vi "myRIO_BRig_RT__Case_Exp_State_initTrial_LC_ENL1.vi"(6 "input_dataTrial":u16[][](array[numeric]), 7 "input_spout":enum16{"Left", "Right"}(ring), 9 "input_dataBlock":u16[][](array[numeric]), 10 "input_dataLC":u16[](array[numeric]), 11 "input_dataCurrent":u16[](array[numeric])) -> (2 "output_LC__ENL1":bool, 3 "output_LC_led__ENL1":bool, 4 "output_dataTrial":u16[][](array[numeric]), 5 "output_dataCurrent":u16[](array[numeric]))   [LabVIEW 2014]
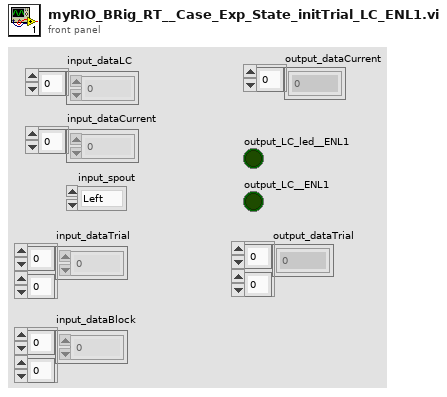
[diagram p1: front panel]
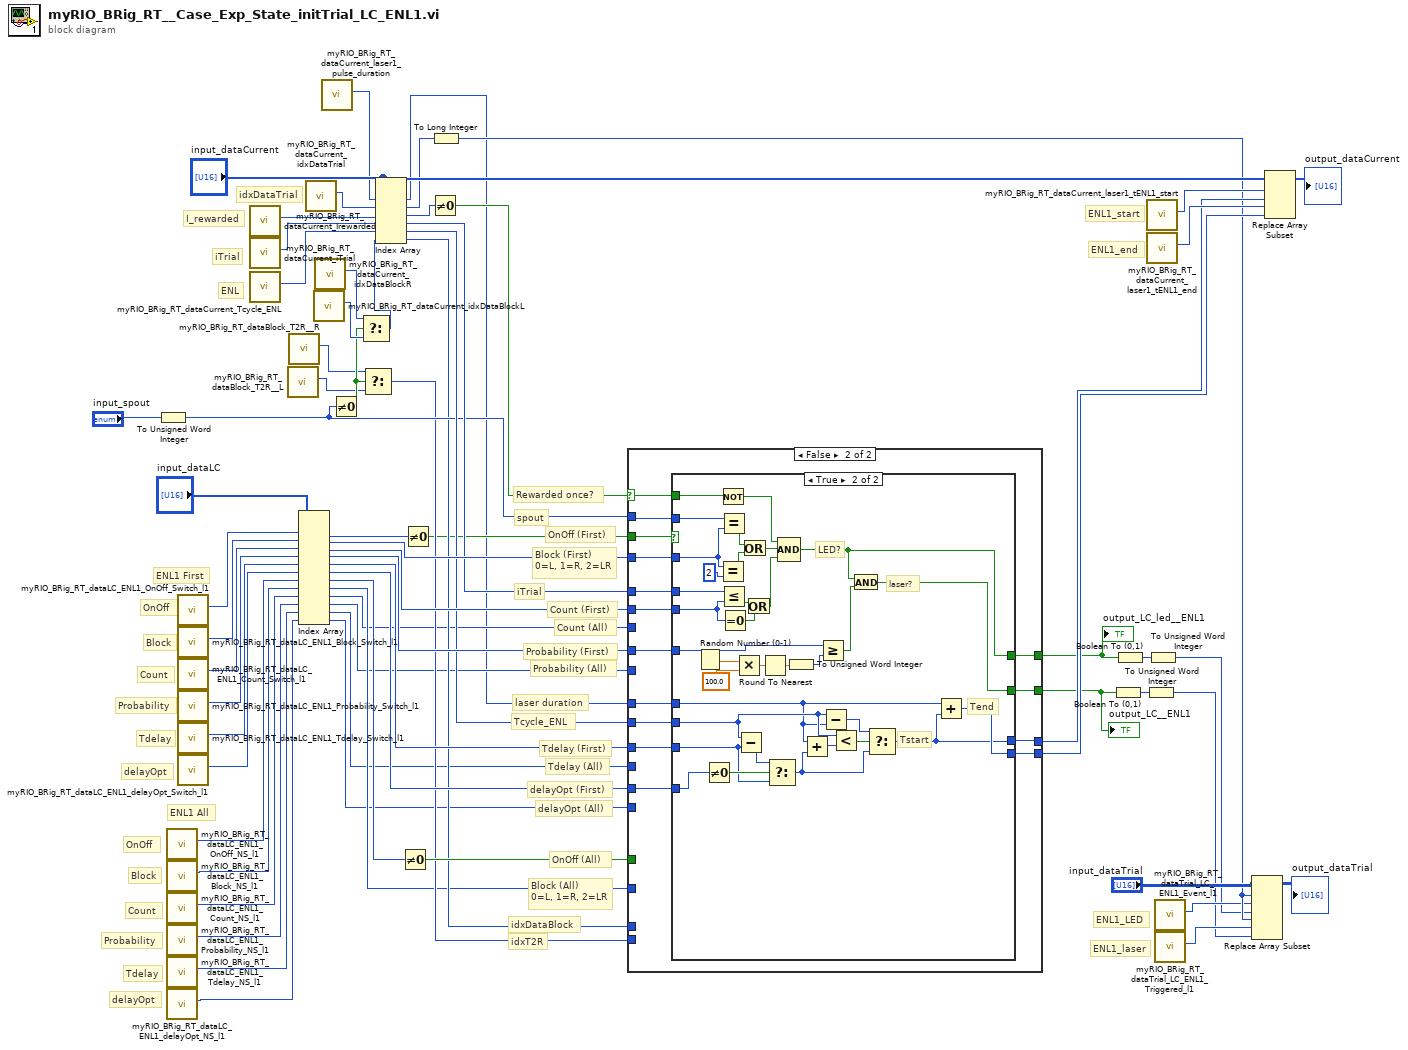
[diagram p0: block diagram]
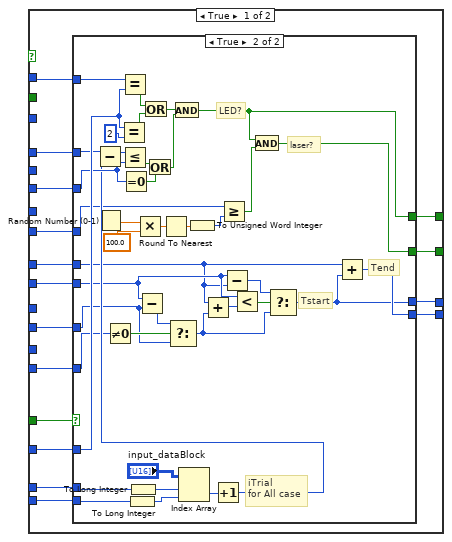
[diagram p2: hidden frame]
diagram:
  # "delayOpt (All)"
  # "Tdelay (All)"
  # "Probability (All)"
  # "Count (All)"
  # "Block (All)\n0=L, 1=R, 2=LR"
  # "idxT2R"
  # "idxDataBlock"
  # "OnOff (All)"
  # "delayOpt"
  # "Count"
  # "Tdelay"
  # "Probability"
  # "OnOff"
  # "Block"
  # "ENL1 All"
  # "Tdelay (First)"
  # "delayOpt (First)"
  # "Tcycle_ENL"
  # "laser duration"
  # "Probability (First)"
  # "Count (First)"
  # "iTrial"
  # "Block (First)\n0=L, 1=R, 2=LR"
  # "spout"
  # "Rewarded once?"
  # "OnOff (First)"
  # "iTrial"
  # "ENL1_LED"
  # "ENL1_laser"
  # "idxDataTrial"
  # "ENL1_end"
  # "ENL1_start"
  # "delayOpt"
  # "ENL"
  # "Tdelay"
  # "I_rewarded"
  # "ENL1 First"
  # "Probability"
  # "Count"
  # "Block"
  # "OnOff"
  n1 = To Unsigned Word Integer(number="input_spout") -> (unsigned 16bit integer=w24:u16)
  n2 = call "myRIO_BRig_RT_dataLC_ENL1_OnOff_NS_l1.vi"() -> ("output_ENL1_OnOff_NS_l1"=w10:i32)  [unwired: 11 in]
  n3 = call "myRIO_BRig_RT_dataLC_ENL1_Block_NS_l1.vi"() -> ("output_ENL1_All_Block"=w9:i32)  [unwired: 11 in]
  n4 = call "myRIO_BRig_RT_dataLC_ENL1_Count_NS_l1.vi"() -> ("output_ENL1_Count_NS_l1"=w8:i32)  [unwired: 11 in]
  n5 = call "myRIO_BRig_RT_dataLC_ENL1_Probability_NS_l1.vi"() -> ("output_ENL1_Probability_NS_l1"=w7:i32)  [unwired: 11 in]
  n6 = call "myRIO_BRig_RT_dataLC_ENL1_Tdelay_NS_l1.vi"() -> ("output_ENL1_Tdelay_NS_l1"=w6:i32)  [unwired: 11 in]
  n7 = call "myRIO_BRig_RT_dataLC_ENL1_delayOpt_NS_l1.vi"() -> ("output_ENL1_delayOpt_NS_l1"=w5:i32)  [unwired: 11 in]
  n8 = call "myRIO_BRig_RT_dataLC_ENL1_OnOff_Switch_l1.vi"() -> ("output_ENL1_OnOff_Switch_l1"=w64:i32)  [unwired: 11 in]
  n9 = call "myRIO_BRig_RT_dataLC_ENL1_Block_Switch_l1.vi"() -> ("output_ENL1_Block_Switch_l1"=w63:i32)  [unwired: 11 in]
  n10 = call "myRIO_BRig_RT_dataLC_ENL1_Count_Switch_l1.vi"() -> ("output_ENL1_Count_Switch_l1"=w62:i32)  [unwired: 11 in]
  n11 = call "myRIO_BRig_RT_dataLC_ENL1_Probability_Switch_l1.vi"() -> ("output_ENL1_Probability_Switch_l1"=w61:i32)  [unwired: 11 in]
  n12 = call "myRIO_BRig_RT_dataLC_ENL1_Tdelay_Switch_l1.vi"() -> ("output_ENL1_Tdelay_Switch_l1"=w53:i32)  [unwired: 11 in]
  n13 = call "myRIO_BRig_RT_dataLC_ENL1_delayOpt_Switch_l1.vi"() -> ("output_ENL1_delayOpt_Switch_l1"=w51:i32)  [unwired: 11 in]
  n14 = call "myRIO_BRig_RT_dataCurrent_Irewarded.vi"() -> ("output_I_rewarded"=w54:i32)  [unwired: 11 in]
  n15 = call "myRIO_BRig_RT_dataCurrent_iTrial.vi"() -> ("output_iTrial"=w28:i32)  [unwired: 11 in]
  n16 = call "myRIO_BRig_RT_dataCurrent_Tcycle_ENL.vi"() -> ("output_ENL"=w30:i32)  [unwired: 11 in]
  n17 = call "myRIO_BRig_RT_dataBlock_T2R__L.vi"() -> ("output_T2R__L"=w18:i32)  [unwired: 11 in]
  n18 = call "myRIO_BRig_RT_dataBlock_T2R__R.vi"() -> ("output_T2R__R"=w19:i32)  [unwired: 11 in]
  n19 = Index Array(array="input_dataLC", index #1=w64, index #2=w63, index #3=w62, index #4=w61, index #5=w53, index #6=w51, index #7=w10, index #8=w9, index #9=w8, index #10=w7, index #11=w6, index #12=w5) -> (element #1=w60:u16, element #2=w57:u16, element #3=w58:u16, element #4=w59:u16, element #5=w52:u16, element #6=w50:u16, element #7=w26:u16, element #8=w15:u16, element #9=w14:u16, element #10=w13:u16, element #11=w12:u16, element #12=w11:u16)
  n20 = call "myRIO_BRig_RT_dataCurrent_idxDataTrial.vi"() -> ("output_idxDataTrial"=w37:i32)  [unwired: 11 in]
  n21 = call "myRIO_BRig_RT_dataCurrent_idxDataBlockL.vi"() -> ("output_idxDataBlock__L"=w23:i32)  [unwired: 11 in]
  n22 = call "myRIO_BRig_RT_dataCurrent_idxDataBlockR.vi"() -> ("output_idxDataBlock__R"=w22:i32)  [unwired: 11 in]
  n23 = call "myRIO_BRig_RT_dataCurrent_laser1_pulse_duration.vi"() -> ("output_laser1_pulse_duration"=w2:i32)  [unwired: 11 in]
  n24 = Not Equal To 0?(x=w24) -> (x != 0?=w20:bool)
  n25 = Select(t=w22, s=w20, f=w23) -> (s? t:f=w21:i32)
  n26 = Select(t=w19, s=w20, f=w18) -> (s? t:f=w16:i32)
  n27 = Index Array(array="input_dataCurrent", index #1=w2, index #2=w37, index #3=w54, index #4=w28, index #5=w30, index #6=w21) -> (element #1=w1:u16, element #2=w36:u16, element #3=w55:u16, element #4=w27:u16, element #5=w29:u16, element #6=w17:u16)
  n28 = Not Equal To 0?(x=w26) -> (x != 0?=w25:bool)
  n29 = Not Equal To 0?(x=w60) -> (x != 0?=w3:bool)
  n30 = Not Equal To 0?(x=w55) -> (x != 0?=w4:bool)
  n31 = To Long Integer(number=w36) -> (32bit integer=w35:i32)
  n32 = case shown="False" w4 {
    selector: w4 -> [_ w123]
    tunnel: w57 -> [_ w135]
    tunnel: w58 -> [_ w126]
    tunnel: w59 -> [_ w133]
    tunnel: [w78 w131] -> w40
    tunnel: [w79 w132] -> w42
    tunnel: w24 -> [w81 w136]
    tunnel: w52 -> [_ w128]
    tunnel: w50 -> [_ w129]
    tunnel: w29 -> [w74 w125]
    tunnel: w1 -> [w75 w124]
    tunnel: [w76 w127] -> w45
    tunnel: [w77 w130] -> w44
    tunnel: w27 -> [w80 w134]
    tunnel: w25 -> [w66 _]
    tunnel: w16 -> [w73 _]
    tunnel: w17 -> [w72 _]
    tunnel: w15 -> [w71 _]
    tunnel: w14 -> [w70 _]
    tunnel: w13 -> [w69 _]
    tunnel: w12 -> [w68 _]
    tunnel: w11 -> [w67 _]
    tunnel: w3 -> [_ w122]
    frame True {
      n33 = case shown="True" w66 {
        tunnel: w81 -> [_ w120]
        tunnel: w80 -> [_ w91]
        tunnel: [_ w82] -> w79
        tunnel: [_ w111] -> w78
        tunnel: [_ w105] -> w77
        tunnel: [_ w104] -> w76
        tunnel: w75 -> [_ w85]
        tunnel: w74 -> [_ w86]
        tunnel: w73 -> [_ w97]
        tunnel: w72 -> [_ w99]
        tunnel: w71 -> [_ w94]
        tunnel: w70 -> [_ w93]
        tunnel: w69 -> [_ w89]
        tunnel: w68 -> [_ w88]
        tunnel: w67 -> [_ w87]
        frame False {
        }
        frame True {
          # "iTrial\nfor All case"
          # "Tend"
          # "Tstart"
          # "laser?"
          # "LED?"
          n34 = Random Number (0-1)() -> (number: 0 to 1=w117:dbl)
          n35 = Not Equal To 0?(x=w87) -> (x != 0?=w110:bool)
          n36 = Equal?(x=w94, y=u16 2) -> (x = y?=w118:bool)
          n37 = Equal?(x=w120, y=w94) -> (x = y?=w119:bool)
          n38 = Equal To 0?(x=w93) -> (x = 0?=w101:bool)
          n39 = To Long Integer(number=w97) -> (32bit integer=w96:i32)
          n40 = To Long Integer(number=w99) -> (32bit integer=w98:i32)
          n41 = Multiply(x=w117, y=100.0) -> (x*y=w116:dbl)
          n42 = Subtract(x=w86, y=w88) -> (x-y=w109:u16)
          n43 = Or(x=w119, y=w118) -> (x .or. y?=w84:bool)
          n44 = Round To Nearest(number=w116) -> (nearest integer value=w115:dbl)
          n45 = Select(t=w109, s=w110, f=w88) -> (s? t:f=w103:u16)
          n46 = Index Array(array="input_dataBlock", index (row)=w98, index (col)=w96) -> (element=w95:u16)
          n47 = To Unsigned Word Integer(number=w115) -> (unsigned 16bit integer=w113:u16)
          n48 = Add(x=w85, y=w103) -> (x+y=w108:u16)
          n49 = Increment(x=w95) -> (x+1=w92:u16)
          n50 = Subtract(x=w91, y=w92) -> (x-y=w90:u16)
          n51 = Less Or Equal?(x=w90, y=w93) -> (x <= y?=w102:bool)
          n52 = Or(x=w102, y=w101) -> (x .or. y?=w83:bool)
          n53 = And(x=w84, y=w83) -> (x .and. y?=w82:bool)
          n54 = Greater Or Equal?(x=w89, y=w113) -> (x >= y?=w112:bool)
          n55 = Subtract(x=w86, y=w85) -> (x-y=w106:u16)
          n56 = Less?(x=w86, y=w108) -> (x < y?=w107:bool)
          n57 = And(x=w82, y=w112) -> (x .and. y?=w111:bool)
          n58 = Select(t=w106, s=w107, f=w103) -> (s? t:f=w104:u16)
          n59 = Add(x=w85, y=w104) -> (x+y=w105:u16)
        }
      }
    }
    frame False {
      n60 = case shown="True" w122 {
        tunnel: w136 -> [_ w169]
        tunnel: w135 -> [_ w168]
        tunnel: w134 -> [_ w167]
        tunnel: w133 -> [_ w160]
        tunnel: [_ w155] -> w132
        tunnel: [_ w154] -> w131
        tunnel: [_ w148] -> w130
        tunnel: w129 -> [_ w147]
        tunnel: w128 -> [_ w146]
        tunnel: [_ w145] -> w127
        tunnel: w126 -> [_ w143]
        tunnel: w125 -> [_ w139]
        tunnel: w124 -> [_ w138]
        tunnel: w123 -> [_ w137]
        frame False {
        }
        frame True {
          # "Tend"
          # "Tstart"
          # "laser?"
          # "LED?"
          n61 = Random Number (0-1)() -> (number: 0 to 1=w164:dbl)
          n62 = Not Equal To 0?(x=w147) -> (x != 0?=w153:bool)
          n63 = Not(x=w137) -> (.not. x?=w158:bool)
          n64 = Equal?(x=w168, y=u16 2) -> (x = y?=w165:bool)
          n65 = Equal?(x=w169, y=w168) -> (x = y?=w166:bool)
          n66 = Less Or Equal?(x=w167, y=w143) -> (x <= y?=w142:bool)
          n67 = Equal To 0?(x=w143) -> (x = 0?=w141:bool)
          n68 = Multiply(x=w164, y=100.0) -> (x*y=w163:dbl)
          n69 = Subtract(x=w139, y=w146) -> (x-y=w152:u16)
          n70 = Or(x=w166, y=w165) -> (x .or. y?=w157:bool)
          n71 = Or(x=w142, y=w141) -> (x .or. y?=w140:bool)
          n72 = Round To Nearest(number=w163) -> (nearest integer value=w162:dbl)
          n73 = Select(t=w152, s=w153, f=w146) -> (s? t:f=w144:u16)
          n74 = Compound Arithmetic op=AND(w158, w157, w140) -> (w155:bool)
          n75 = To Unsigned Word Integer(number=w162) -> (unsigned 16bit integer=w159:u16)
          n76 = Add(x=w138, y=w144) -> (x+y=w151:u16)
          n77 = Greater Or Equal?(x=w160, y=w159) -> (x >= y?=w156:bool)
          n78 = Subtract(x=w139, y=w138) -> (x-y=w149:u16)
          n79 = Less?(x=w139, y=w151) -> (x < y?=w150:bool)
          n80 = And(x=w155, y=w156) -> (x .and. y?=w154:bool)
          n81 = Select(t=w149, s=w150, f=w144) -> (s? t:f=w145:u16)
          n82 = Add(x=w138, y=w145) -> (x+y=w148:u16)
        }
      }
    }
  }
  "output_LC__ENL1" <- w40
  "output_LC_led__ENL1" <- w42
  n83 = Boolean To (0,1)(Boolean=w40) -> (0, 1=w41:i16)
  n84 = Boolean To (0,1)(Boolean=w42) -> (0, 1=w43:i16)
  n85 = To Unsigned Word Integer(number=w41) -> (unsigned 16bit integer=w31:u16)
  n86 = call "myRIO_BRig_RT_dataCurrent_laser1_tENL1_start.vi"() -> ("output_laser1_tENL1_start"=w47:i32)  [unwired: 11 in]
  n87 = call "myRIO_BRig_RT_dataCurrent_laser1_tENL1_end.vi"() -> ("output_laser1_tENL1_end"=w46:i32)  [unwired: 11 in]
  n88 = To Unsigned Word Integer(number=w43) -> (unsigned 16bit integer=w32:u16)
  n89 = call "myRIO_BRig_RT_dataTrial_LC_ENL1_Event_l1.vi"() -> ("output_LC_ENL1_Event_l1"=w34:i32)  [unwired: 11 in]
  n90 = call "myRIO_BRig_RT_dataTrial_LC_ENL1_Triggered_l1.vi"() -> ("output_LC_ENL1_Triggered_l1"=w33:i32)  [unwired: 11 in]
  n91 = Replace Array Subset(array="input_dataTrial", new element #1=w32, index (row) #1=w35, index (col) #1=w34, new element #2=w31, index (row) #2=w35, index (col) #2=w33) -> (→"output_dataTrial":u16[][])
  n92 = Replace Array Subset(array="input_dataCurrent", new element #1=w45, index #1=w47, new element #2=w44, index #2=w46) -> (→"output_dataCurrent":u16[])
